vi "Register For Events.vi"(8 "error in (no error)":errorcluster, 10 "Events To Register":T2[](array[typedef]), 11 "Session in":refnum<class "Plugin Session.lvclass">) -> (0 "error out":errorcluster, 2 "Event Refnum":T1, 3 "Session out":refnum<class "Plugin Session.lvclass">)   [LabVIEW 2023, in "InstrumentStudio Plugin SDK.lvlib" / "Plugin Session.lvclass"]
doc: "Call this VI to let the framework know which events you want to get notifications for. Only pass in events that you are going to handle in your event structure. There are two events available - Project Saved and Stop All Outputs.\n\nProject Saved\nThis event is fired when the path of the Project changes. It passes event data for the updated project path and a Completion Id. The user must call Notify Event Complete with this Completion Id to let the framework know its processing is complete. Failure to do this will result in a hang.\n\nStop All Outputs\nThe Stop All Outputs event is fired when the 'Stop all outputs' button is pressed on the document toolbar. It notifies the plugin that it should cease sending output data to any external devices."
uses:
  Plugin Session.lvclass
  Plugin Events Enum.ctl
  Event Registration Refnum.ctl
  Plugin Events.ctl
  Plugin Session.lvclass/Plugin Session.ctl
  Read Session Id.vi
  Read Plugin Events.vi
  Read Event Refnum.vi
  NationalInstruments.VIHost.Interop.dll
  InstrumentStudio Plugin SDK.lvlib
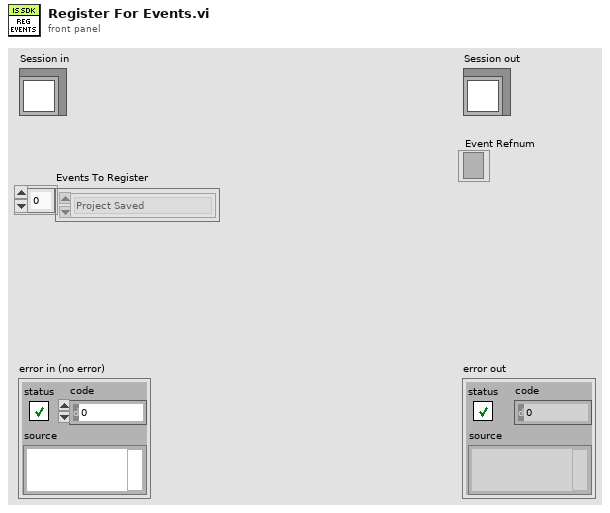
[diagram p1: front panel]
types:
  T1 = typedef "InstrumentStudio Plugin SDK.lvlib/Event Registration Refnum.ctl" = refnum<event-registration>
  T2 = typedef "InstrumentStudio Plugin SDK.lvlib/Plugin Events Enum.ctl" = enum16{"Shutdown", "Project Saved", "Stop All Outputs"}
  T3 = typedef "InstrumentStudio Plugin SDK.lvlib/Plugin Events.ctl" = cluster{"Shutdown":refnum<user-event>, "Project Saved":refnum<user-event>, "Stop All Outputs":refnum<user-event>}
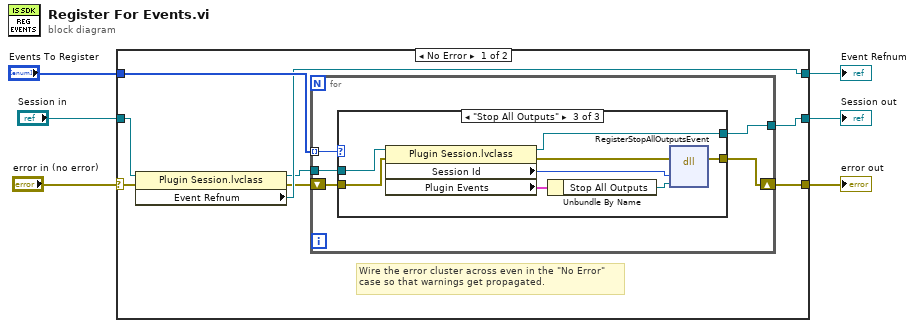
[diagram p0: block diagram]
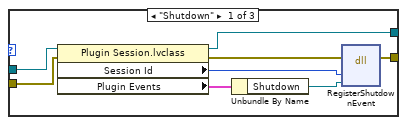
[diagram p2: hidden frame]
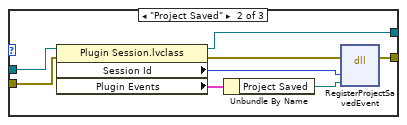
[diagram p3: hidden frame]
diagram:
  n1 = case shown="No Error" "error in (no error)" {
    selector: "error in (no error)" -> [w9 w45]
    tunnel: [w13 w45] -> w5
    tunnel: [w7 w44] -> w3
    tunnel: "Session in" -> [w11 w44]
    tunnel: "Events To Register" -> [w14 _]
    tunnel: [w12 _] -> w1
    frame No Error {
      # "Wire the error cluster across even in the \"No Error\"\ncase so that warnings get propagated."
      n2 = property class="Plugin Session.lvclass"(reference=w11, error in=w9) -> (reference out=w10:refnum<class "Plugin Session.lvclass">, error out=w8:errorcluster, "Event Refnum"=w12:T1)
      n3 = for {
        tunnel: w14 -> [w19] mode=indexing
        tunnel: w10 -> [w18]
        shift-right: [w16] -> w13
        shift-left: w8 -> [w17]
        tunnel: [w15] -> w7
        n4 = case shown="\"Stop All Outputs\"" w19 {
          tunnel: w18 -> [w22 w32 w39]
          tunnel: w17 -> [w23 w31 w38]
          tunnel: [w20 w29 w37] -> w16
          tunnel: [w21 w28 w36] -> w15
          frame "Shutdown" {
            n5 = property class="Plugin Session.lvclass"(reference=w22, error in=w23) -> (reference out=w21:refnum<class "Plugin Session.lvclass">, error out=w27:errorcluster, "Session Id"=w24:u64, "Plugin Events"=w25:T3)
            n6 = Unbundle By Name(w25) -> ("Shutdown"=w26:refnum<user-event>)
            n7 = dll-call lib="C:/Users/nmurphy/Downloads/InstrumentStudio_LabVIEW_Plugins/LabVIEW/ExampleProject/PluginSDK/NationalInstruments.VIHost.Interop.dll" fn="RegisterShutdownEvent"(error in=w27, "hostId"=w24, "eventRef"=w26) -> (error out=w20:errorcluster)  [unwired: 5 in, 1 out]
          }
          frame "Project Saved" {
            n8 = property class="Plugin Session.lvclass"(reference=w32, error in=w31) -> (reference out=w28:refnum<class "Plugin Session.lvclass">, error out=w30:errorcluster, "Session Id"=w35:u64, "Plugin Events"=w34:T3)
            n9 = Unbundle By Name(w34) -> ("Project Saved"=w33:refnum<user-event>)
            n10 = dll-call lib="C:/Users/nmurphy/Downloads/InstrumentStudio_LabVIEW_Plugins/LabVIEW/ExampleProject/PluginSDK/NationalInstruments.VIHost.Interop.dll" fn="RegisterProjectSavedEvent"(error in=w30, "hostId"=w35, "projectSavedEventRef"=w33) -> (error out=w29:errorcluster)  [unwired: 5 in, 1 out]
          }
          frame "Stop All Outputs" {
            n11 = property class="Plugin Session.lvclass"(reference=w39, error in=w38) -> (reference out=w36:refnum<class "Plugin Session.lvclass">, error out=w40:errorcluster, "Session Id"=w43:u64, "Plugin Events"=w42:T3)
            n12 = Unbundle By Name(w42) -> ("Stop All Outputs"=w41:refnum<user-event>)
            n13 = dll-call lib="C:/Users/nmurphy/Downloads/InstrumentStudio_LabVIEW_Plugins/LabVIEW/ExampleProject/PluginSDK/NationalInstruments.VIHost.Interop.dll" fn="RegisterStopAllOutputsEvent"(error in=w40, "hostId"=w43, "eventRef"=w41) -> (error out=w37:errorcluster)  [unwired: 5 in, 1 out]
          }
        }
      }
    }
    frame Error {
    }
  }
  "error out" <- w5
  "Session out" <- w3
  "Event Refnum" <- w1
